vi "Hypergeometric Random.vi"(6 "seed":i32=-1, 7 "reset":bool, 8 "n":i32=20, 9 "k":i32=30, 10 "M":i32=100, 11 "samples":i32=128) -> (0 "error":i32, 3 "hypergeometric random data":i32[](array[numeric]))   [LabVIEW 2017, in "NI_Gmath.lvlib"]
doc: "Generates random values from a variate X, where X describes the selected distribution type. You must manually select the polymorphic instance to use."
uses:
  NI_Gmath.lvlib
panel:
  # "Hypergeometric Random"
  # "size of population"
  # "items"
  # "samples drawn"
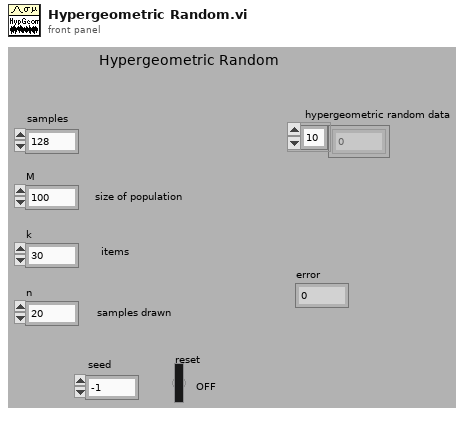
[diagram p1: front panel]
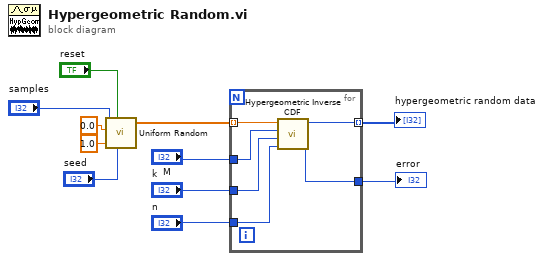
[diagram p0: block diagram]
diagram:
  n1 = call "Uniform Random.vi"("seed"="seed", "reset"="reset", "xmax"=1.0, "xmin"=0.0, "samples"="samples") -> ("uniform random data"=w9:dbl[])  [unwired: 5 in, 1 out]
  n2 = for {
    tunnel: [w17] -> w7 mode=indexing
    tunnel: [w16] -> w6
    tunnel: w9 -> [w15] mode=indexing
    tunnel: "M" -> [w14]
    tunnel: "k" -> [w13]
    tunnel: "n" -> [w12]
    n3 = call "Hypergeometric Inverse CDF.vi"("n"=w12, "k"=w13, "M"=w14, "cdf(x)"=w15) -> ("error"=w16:i32, "x"=w17:i32)  [unwired: 6 in]
  }
  "hypergeometric random data" <- w7
  "error" <- w6
